vi "pcbPositioning_working.vi"() -> ()   [LabVIEW 2015]
uses:
  GlobalPath.vi
  GlobalData.vi
  GlobalVi.vi
panel:
  out "error out 2":errorcluster
  out "file or folder exists?":bool
  out "error out":errorcluster
  in  "?":bool
  in  "Done ?":bool
  out "Test type":string="Table"
  out "PanelName":string="RSS1-0-0001"
  in  "ptfe 2":bool caption="Position the 12 PTFE pins in their dedicated holes on the reference plates"
  in  "PCB 6":bool caption="Position the PCBs on the reference plates starting from the largest one"
  in  "visual 4":bool caption="Check the PCBs for possible defects"
  in  "visual 3":bool caption="Verify that the interconnections and pin inserts alligned to the FEB are mounted in position"
  in  "Table or Stiffback?":bool
  out "PcbFirstPart":string
  in  "stop 2":bool
  in  "Save the IDs in the database? Leave the DB open when done":bool
  in  "Fill database with all 5 PCB IDs? \nTo do this click on the PCB tab, start filling from tab 1 (1 tab per PCB), fill the \"Enter Serial/Get From DB\" box, click \"check_db\"\nThen click on the box \"Position\" ands select the PCB postition (1-5 for table and stiff1-stiff5 for the stiffback)\nThen press Add/Update \"Entry\"":bool
  in  "PCB 1":string
  in  "PCB 2":string
  in  "PCB 3":string
  in  "PCB 4":string
  in  "PCB 5":string
  # "PCB positioning on table/stiffback"
  # "(True if Table)"
  # "PCB ID recording"
  # "Fill each box with the correct ID last four digits, choose table or stiffback and press SAVE"
  # "PCB identifying through the database"
  # "Scan the ID of each of the 5 PCBs and associate them with the panel"
  # "(If the database window is closed, then click here  -->                 and load the correct panel this way: Add>Add then from the list choose \"Readout\" and then Start\n                                                                                                                                                                                                                     Choose the correct ID and click \"Start building panel\")"
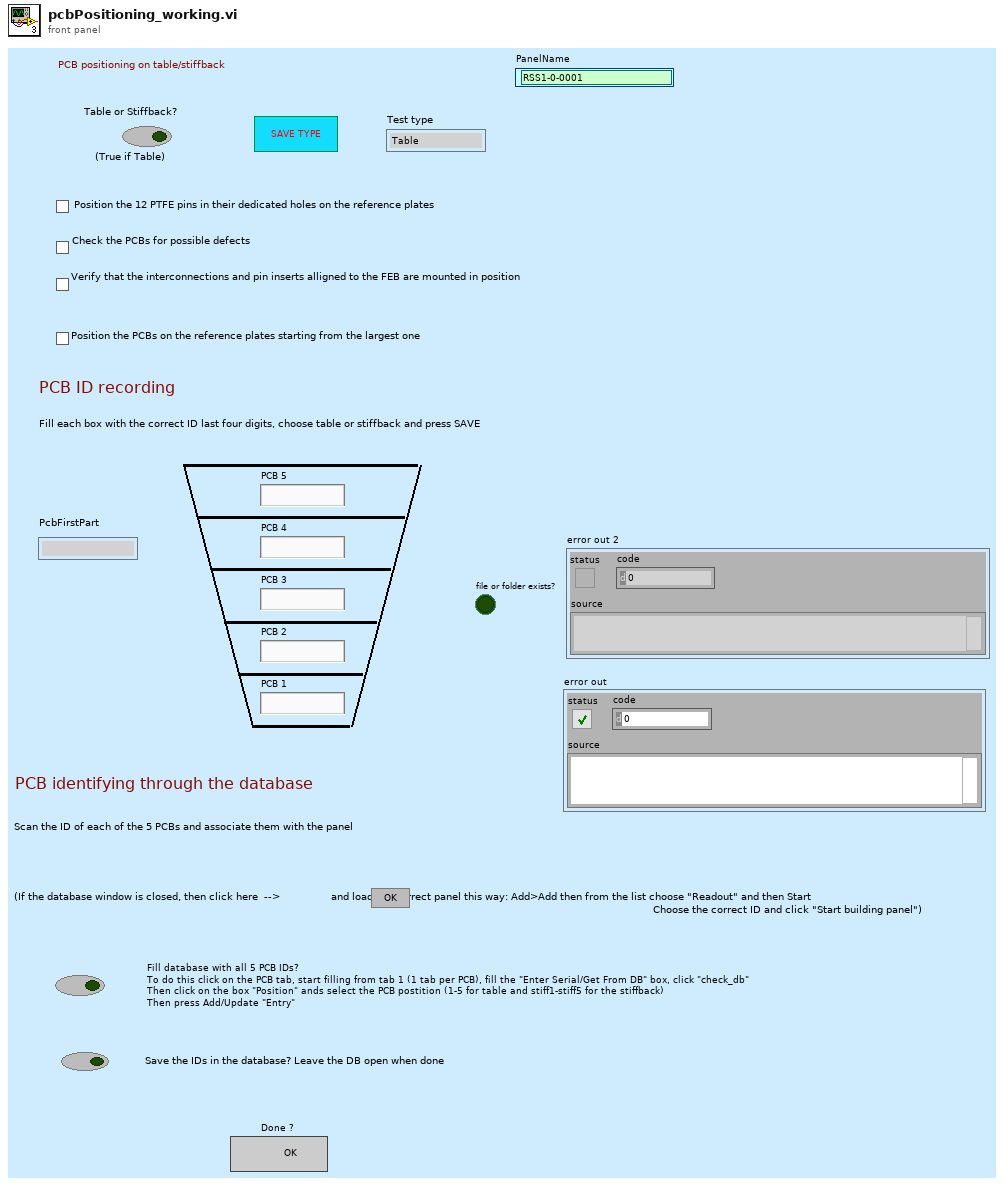
[diagram p1: front panel]
types:
  T1 = enum16{"open", "replace", "create", "open or create", "replace or create", "replace or create with confirmation"}
  T2 = enum32{"Bad", "Idle", "Run top level", "Running"}
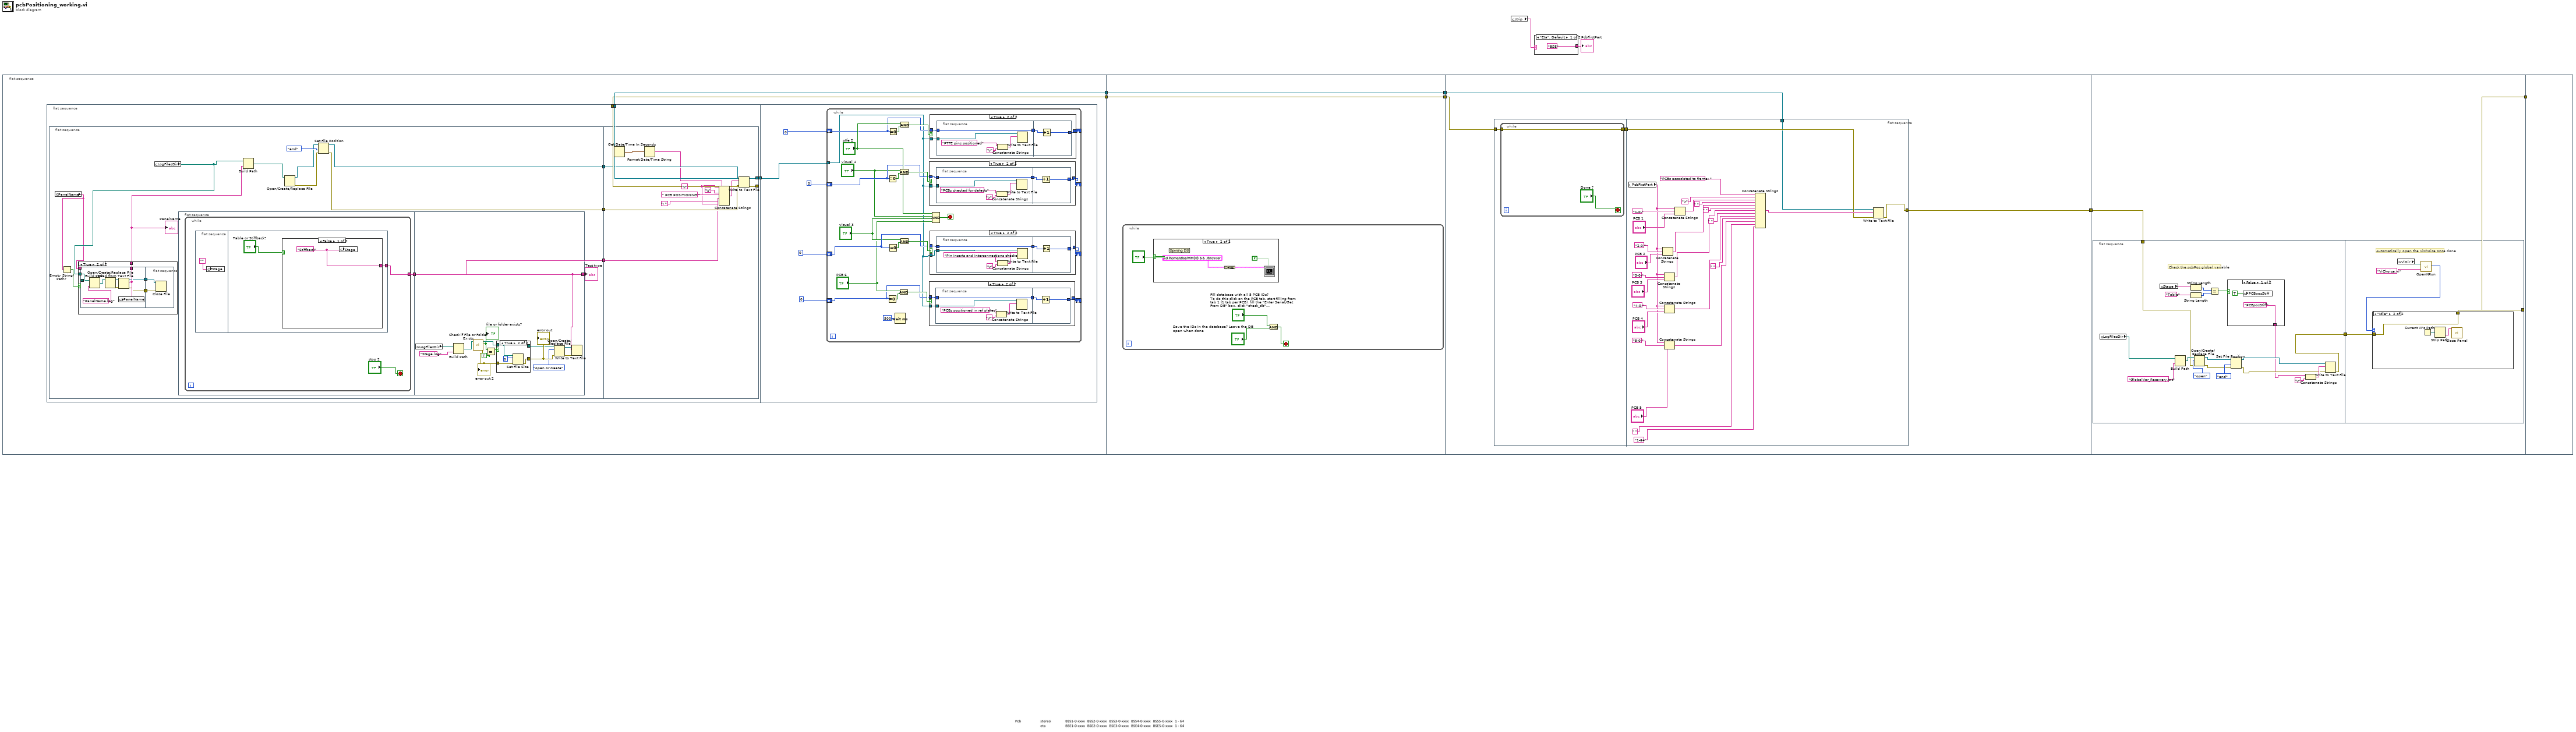
[diagram p0: block diagram]
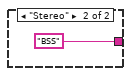
[diagram p2: hidden frame]
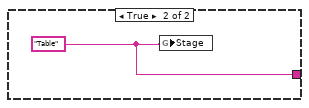
[diagram p3: hidden frame]
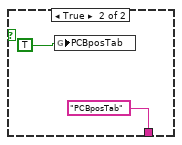
[diagram p11: hidden frame]
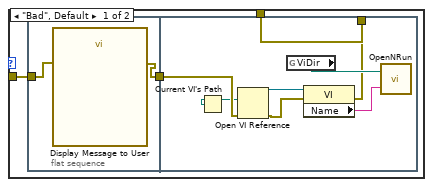
[diagram p12: hidden frame]
diagram:
  n1 = flat-sequence {
    tunnel: [w10] -> w8
    tunnel: [w9] -> w7
    tunnel: w8 -> [w161]
    tunnel: [w161] -> w2
    tunnel: w7 -> [w160]
    tunnel: [w160] -> w1
    tunnel: w2 -> [w166]
    tunnel: [w167] -> w5
    tunnel: w1 -> [w169]
    tunnel: [w204] -> w6
    tunnel: w5 -> [w202]
    tunnel: w6 -> [_]
    frame #0 {
      n2 = flat-sequence {
        tunnel: [w15] -> w11
        tunnel: [w15] -> w10
        tunnel: [w14] -> w9
        tunnel: w11 -> [w88]
        frame #0 {
          n3 = flat-sequence {
            tunnel: [w23] -> w16
            tunnel: [w25] -> w13
            tunnel: [w22] -> w12
            tunnel: w16 -> [w80]
            tunnel: [w79] -> w15
            tunnel: [w78] -> w14
            tunnel: w13 -> [w77]
            tunnel: w12 -> [w74]
            frame #0 {
              n4 = global read "GlobalData.vi" "PanelName"() -> (w19:string)
              n5 = Empty String/Path?(string/path=w19) -> (empty?=w21:bool)
              n6 = global read "GlobalPath.vi" "LogFilesDir"() -> (w20:path)
              n7 = case shown="True" w21 {
                tunnel: w20 -> [_ w61]
                tunnel: [w57 w60] -> w18
                tunnel: w19 -> [w57 _]
                frame False {
                }
                frame True {
                  n8 = flat-sequence {
                    tunnel: w61 -> [w69]
                    tunnel: [w64] -> w60
                    tunnel: [w63] -> w59
                    tunnel: [w62] -> w58
                    tunnel: w59 -> [w71]
                    tunnel: w58 -> [w70]
                    frame #0 {
                      n9 = Build Path(base path=w69, name or relative path="PanelName.log") -> (appended path=w68:path)
                      n10 = Open/Create/Replace File(file path (use dialog)=w68) -> (refnum out=w65:refnum<file>, error out=w66:errorcluster)  [unwired: 5 in, 1 out]
                      n11 = Read from Text File(file (use dialog)=w65, error in=w66) -> (refnum out=w62:refnum<file>, text=w64:string, error out=w63:errorcluster)  [unwired: 2 in, 1 out]
                      n12 = global write "GlobalData.vi" "PanelName"(w64) -> ()
                    }
                    frame #1 {
                      n13 = Close File(refnum=w70, error in=w71) -> ()  [unwired: 2 out]
                    }
                  }
                }
              }
              "PanelName" <- w18
              n14 = flat-sequence {
                tunnel: [w29] -> w17
                tunnel: [w37] -> w22
                tunnel: w17 -> [w37]
                frame #0 {
                  n15 = while {
                    tunnel: [w30] -> w29
                    stop <- "stop 2" stop-if-true
                    n16 = flat-sequence {
                      tunnel: [w33] -> w30
                      frame #0 {
                        n17 = global write "GlobalData.vi" "Stage"("") -> ()
                      }
                      frame #1 {
                        n18 = case shown="False" "Table or Stiffback?" {
                          tunnel: [w35 w36] -> w33
                          frame False {
                            w35 = "Stiffback"
                            n19 = global write "GlobalData.vi" "Stage"(w35) -> ()
                          }
                          frame True {
                            w36 = "Table"
                            n20 = global write "GlobalData.vi" "Stage"(w36) -> ()
                          }
                        }
                      }
                    }
                  }
                }
                frame #1 {
                  n21 = global read "GlobalPath.vi" "LogFilesDir"() -> (w45:path)
                  n22 = Build Path(base path=w45, name or relative path="Stage.log") -> (appended path=w44:path)
                  n23 = call <vilib>:"Check if File or Folder Exists.vi"("path"=w44) -> ("error out"=w40:errorcluster, "file or folder exists?"=w43:bool, "dup path"=w50:path)  [unwired: 8 in]
                  "file or folder exists?" <- w43
                  "error out 2" <- w40
                  n24 = Equal?(x=w43, y=TRUE) -> (x = y?=w39:bool)
                  n25 = case shown="True" w39 {
                    tunnel: w50 -> [w52 w55]
                    tunnel: [w52 w55] -> w41
                    tunnel: [w51 w54] -> w49
                    tunnel: w40 -> [w51 w53]
                    frame False {
                    }
                    frame True {
                      n26 = Set File Size(4:w53, 6:0, 7:w55) -> (0:w54:errorcluster)  [unwired: 1 out]
                    }
                  }
                  "error out" <- w49
                  n27 = Open/Create/Replace File(file path (use dialog)=w41, error in=w49, operation (0:open)=T1."open or create") -> (refnum out=w48:refnum<file>, error out=w47:errorcluster)  [unwired: 3 in, 1 out]
                  n28 = Write to Text File(file (use dialog)=w48, text=w37, error in=w47) -> ()  [unwired: 1 in, 3 out]
                }
              }
              n29 = Build Path(base path=w20, name or relative path=w18) -> (appended path=w28:path)
              n30 = Open/Create/Replace File(file path (use dialog)=w28) -> (refnum out=w24:refnum<file>, error out=w26:errorcluster)  [unwired: 5 in, 1 out]
              n31 = Set File Position(refnum=w24, from (0:start)=enum16{"start", "end", "current"}."end", error in=w26) -> (refnum out=w23:refnum<file>, error out=w25:errorcluster)  [unwired: 1 in]
              "Test type" <- w22
            }
            frame #1 {
              w72 = "\r"
              n32 = Get Date/Time In Seconds() -> (seconds since 1Jan1904=w76:timestamp)
              n33 = Format Date/Time String(seconds (now)=w76) -> (date/time string=w75:string)  [unwired: 2 in]
              n34 = Concatenate Strings(w72, w75, "\t", " PCB POSITIONING ", w74, ": ", w72) -> (w81:string)
              n35 = Write to Text File(file (use dialog)=w80, text=w81, error in=w77) -> (refnum out=w79:refnum<file>, error out=w78:errorcluster)  [unwired: 1 in, 1 out]
            }
          }
        }
        frame #1 {
          n36 = while {
            tunnel: w88 -> [w90]
            shift-right: [w105] -> _
            shift-left: 0 -> [w106]
            shift-right: [w95] -> _
            shift-left: 0 -> [w102]
            shift-right: [w96] -> _
            shift-left: 0 -> [w98]
            shift-right: [w89] -> _
            shift-left: 0 -> [w91]
            stop <- w111 stop-if-true
            n37 = Equal To 0?(x=w91) -> (x = 0?=w94:bool)
            n38 = Equal To 0?(x=w102) -> (x = 0?=w104:bool)
            n39 = Equal To 0?(x=w98) -> (x = 0?=w100:bool)
            n40 = Equal To 0?(x=w106) -> (x = 0?=w109:bool)
            n41 = Wait (ms)(milliseconds to wait=u32 500) -> ()  [unwired: 1 out]
            n42 = And(x="PCB 6", y=w94) -> (x .and. y?=w93:bool)
            n43 = And(x="visual 4", y=w104) -> (x .and. y?=w103:bool)
            n44 = And(x="visual 3", y=w100) -> (x .and. y?=w99:bool)
            n45 = And(x="ptfe 2", y=w109) -> (x .and. y?=w107:bool)
            n46 = case shown="True" w93 {
              tunnel: w90 -> [_ w116]
              tunnel: w91 -> [w112 w114]
              tunnel: [w112 w113] -> w89
              frame False {
              }
              frame True {
                n47 = flat-sequence {
                  tunnel: w116 -> [w118]
                  tunnel: [w117] -> w115
                  tunnel: w114 -> [w117]
                  tunnel: w115 -> [w123]
                  tunnel: [w122] -> w113
                  frame #0 {
                    n48 = Concatenate Strings("PCBs positioned in ref plates", "\r") -> (w121:string)
                    n49 = Write to Text File(file (use dialog)=w118, text=w121) -> ()  [unwired: 2 in, 3 out]
                  }
                  frame #1 {
                    n50 = Increment(x=w123) -> (x+1=w122:i32)
                  }
                }
              }
            }
            n51 = case shown="True" w103 {
              tunnel: w90 -> [_ w140]
              tunnel: w102 -> [w136 w138]
              tunnel: [w136 w137] -> w95
              frame False {
              }
              frame True {
                n52 = flat-sequence {
                  tunnel: w140 -> [w142]
                  tunnel: [w141] -> w139
                  tunnel: w138 -> [w141]
                  tunnel: w139 -> [w147]
                  tunnel: [w146] -> w137
                  frame #0 {
                    n53 = Concatenate Strings("PCBs checked for defects", "\r") -> (w145:string)
                    n54 = Write to Text File(file (use dialog)=w142, text=w145) -> ()  [unwired: 2 in, 3 out]
                  }
                  frame #1 {
                    n55 = Increment(x=w147) -> (x+1=w146:i32)
                  }
                }
              }
            }
            n56 = case shown="True" w99 {
              tunnel: w90 -> [_ w128]
              tunnel: w98 -> [w124 w126]
              tunnel: [w124 w125] -> w96
              frame False {
              }
              frame True {
                n57 = flat-sequence {
                  tunnel: w128 -> [w130]
                  tunnel: [w129] -> w127
                  tunnel: w126 -> [w129]
                  tunnel: w127 -> [w135]
                  tunnel: [w134] -> w125
                  frame #0 {
                    n58 = Concatenate Strings("Pin inserts and interconnections checked", "\r") -> (w133:string)
                    n59 = Write to Text File(file (use dialog)=w130, text=w133) -> ()  [unwired: 2 in, 3 out]
                  }
                  frame #1 {
                    n60 = Increment(x=w135) -> (x+1=w134:i32)
                  }
                }
              }
            }
            n61 = case shown="True" w107 {
              tunnel: w90 -> [_ w152]
              tunnel: w106 -> [w148 w150]
              tunnel: [w148 w149] -> w105
              frame False {
              }
              frame True {
                n62 = flat-sequence {
                  tunnel: w152 -> [w154]
                  tunnel: [w153] -> w151
                  tunnel: w150 -> [w153]
                  tunnel: w151 -> [w159]
                  tunnel: [w158] -> w149
                  frame #0 {
                    n63 = Concatenate Strings("PTFE pins positioned", "\r") -> (w157:string)
                    n64 = Write to Text File(file (use dialog)=w154, text=w157) -> ()  [unwired: 2 in, 3 out]
                  }
                  frame #1 {
                    n65 = Increment(x=w159) -> (x+1=w158:i32)
                  }
                }
              }
            }
            n66 = Compound Arithmetic op=AND("ptfe 2", "visual 4", "visual 3", "PCB 6") -> (w111:bool)
          }
        }
      }
    }
    frame #1 {
      n67 = while {
        stop <- w163 stop-if-true
        n68 = case shown="True" "?" {
          frame False {
          }
          frame True {
          }
        }
        n69 = And(x="Fill database with all 5 PCB IDs? \nTo do this click on the PCB tab, start filling from tab 1 (1 tab per PCB), fill the \"Enter Serial/Get From DB\" box, click \"check_db\"\nThen click on the box \"Position\" ands select the PCB postition (1-5 for table and stiff1-stiff5 for the stiffback)\nThen press Add/Update \"Entry\"", y="Save the IDs in the database? Leave the DB open when done") -> (x .and. y?=w163:bool)
      }
    }
    frame #2 {
      n70 = flat-sequence {
        tunnel: w169 -> [w171]
        tunnel: [w170] -> w168
        tunnel: w168 -> [w176]
        tunnel: [w174] -> w167
        tunnel: w166 -> [w175]
        frame #0 {
          n71 = while {
            tunnel: w171 -> [w172]
            tunnel: [w172] -> w170
            stop <- "Done ?" stop-if-true
          }
        }
        frame #1 {
          n72 = local read "PcbFirstPart"() -> (w177:string)
          n73 = Concatenate Strings(w177, "2-0-", "PCB 2") -> (w187:string)
          n74 = Concatenate Strings(w177, "3-0-", "PCB 3") -> (w185:string)
          n75 = Concatenate Strings(w177, "4-0-", "PCB 4") -> (w183:string)
          n76 = Concatenate Strings(w177, "5-0-", "PCB 5") -> (w181:string)
          n77 = Concatenate Strings(w177, "1-0-", "PCB 1") -> (w189:string)
          n78 = Concatenate Strings("PCBs associated to frame: ", "\r", w189, " ", w187, " ", w185, " ", w183, " ", w181, " ", "1-64") -> (w178:string)
          n79 = Write to Text File(file (use dialog)=w175, text=w178, error in=w176) -> (error out=w174:errorcluster)  [unwired: 1 in, 2 out]
        }
      }
    }
    frame #3 {
      n80 = flat-sequence {
        tunnel: [w208] -> w203
        tunnel: w202 -> [w207]
        tunnel: [w229] -> w204
        tunnel: w203 -> [w228]
        frame #0 {
          # "Check the pcbPos global variable"
          n81 = global read "GlobalPath.vi" "LogFilesDir"() -> (w205:path)
          n82 = global read "GlobalData.vi" "Stage"() -> (w219:string)
          n83 = Build Path(base path=w205, name or relative path="GlobalVar_Recovery.txt") -> (appended path=w217:path)
          n84 = String Length(string=w219) -> (length=w221:i32)
          n85 = String Length(string="Table") -> (length=w222:i32)
          n86 = Open/Create/Replace File(file path (use dialog)=w217, error in=w207, operation (0:open)=T1."open") -> (refnum out=w213:refnum<file>, error out=w214:errorcluster)  [unwired: 3 in, 1 out]
          n87 = Equal?(x=w221, y=w222) -> (x = y?=w223:bool)
          n88 = case shown="False" w223 {
            tunnel: ["PCBposStiff" "PCBposTab"] -> w206
            frame False {
              n89 = global write "GlobalVi.vi" "PCBposStiff"(TRUE) -> ()
            }
            frame True {
              n90 = global write "GlobalVi.vi" "PCBposTab"(TRUE) -> ()
            }
          }
          n91 = Set File Position(refnum=w213, from (0:start)=enum16{"start", "end", "current"}."end", error in=w214) -> (refnum out=w210:refnum<file>, error out=w209:errorcluster)  [unwired: 1 in]
          n92 = Concatenate Strings(w206, "\r") -> (w212:string)
          n93 = Write to Text File(file (use dialog)=w210, text=w212, error in=w209) -> (error out=w208:errorcluster)  [unwired: 1 in, 2 out]
        }
        frame #1 {
          # "Automatically open the ViChoice once done"
          n94 = global read "GlobalPath.vi" "ViDir"() -> (w232:path)
          n95 = call "OpenNRun.vi"("VI name"="ViChoice.vi", "ViDirPath"=w232) -> ("Execution:State"=w231:T2)
          n96 = case shown="\"Idle\"" w231 {
            tunnel: [w235 w245] -> w229
            tunnel: w228 -> [w234 w245]
            frame "Bad", Default {
              n97 = flat-sequence {
                tunnel: w234 -> [w237]
                tunnel: [w236] -> w233
                tunnel: [w240] -> w235
                tunnel: w233 -> [w239]
                frame #0 {
                  n98 = call "Display Message to User"("error in (no error)"=w237) -> ("error out"=w236:errorcluster)  [unwired: 9 in, 1 out]
                }
                frame #1 {
                  n99 = Current VI's Path() -> (path=w238:path)
                  n100 = Open VI Reference(vi path=w238, error in (no error)=w239) -> (vi reference=w244:refnum<vi>, error out=w243:errorcluster)  [unwired: 4 in]
                  n101 = global read "GlobalPath.vi" "ViDir"() -> (w242:path)
                  n102 = property class="VI"(reference=w244, error in=w243) -> (error out=w240:errorcluster, "Name"=w241:string)  [unwired: 1 out]
                  n103 = call "OpenNRun.vi"("VI name"=w241, "ViDirPath"=w242) -> ()  [unwired: 1 out]
                }
              }
            }
            frame "Idle" {
              n104 = Current VI's Path() -> (path=w246:path)
              n105 = Strip Path(path=w246) -> (name=w247:string)  [unwired: 1 out]
              n106 = call <vilib>:"Close Panel.vi"("VI name"=w247) -> ()  [unwired: 10 in, 1 out]
            }
          }
        }
      }
    }
    frame #4 {
    }
  }
  n107 = global read "GlobalData.vi" "strip"() -> (w4:string)
  n108 = case shown="\"Eta\", Default" w4 {
    tunnel: ["BSE" "BSS"] -> w3
    frame "Eta", Default {
    }
    frame "Stereo" {
    }
  }
  "PcbFirstPart" <- w3
